vi "Save Waveform Results to CSV.vi"() -> ()   [LabVIEW 2010]
panel:
  out "error out":errorcluster
  in  "error in":errorcluster
  in  "results file":path=path "C:/Documents and Settings/user/Desktop/Claytons Archive/results.csv"
  in  "Data Files":path[](array[path])=[path "C:/5-01-003 Active Electrode Min Max/Waveform 1 -5 mA", path "C:/5-01-003 Active Electrode Min Max/Waveform 2 -0.02 mA", path "C:/5-01-003 Active Electrode Min Max/Waveform 3 -10 mA", path "C:/5-01-003 Active Electrode Min Max/Waveform 4 3 mA", path "C:/5-01-003 Active Electrode Min Max/Waveform 5 0.02 mA", path "C:/5-01-003 Active Electrode Min Max/Waveform 6 10 mA"]
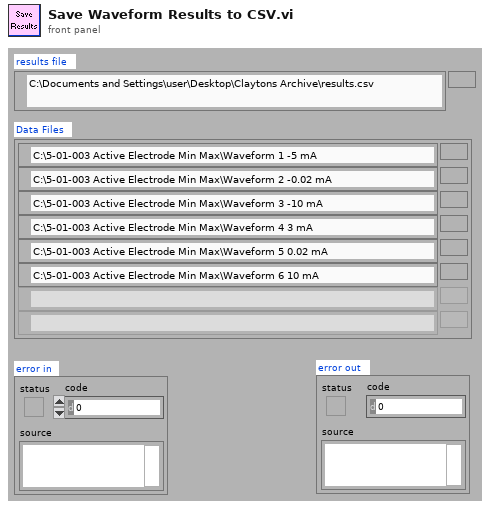
[diagram p1: front panel]
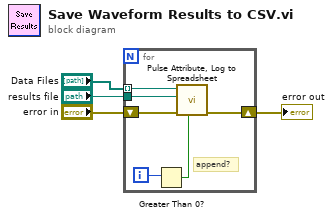
[diagram p0: block diagram]
diagram:
  n1 = for {
    shift-right: [w9] -> w2
    shift-left: "error in" -> [w10]
    tunnel: "Data Files" -> [w8] mode=indexing
    tunnel: "results file" -> [w7]
    i -> [w6]
    # "append?"
    n2 = Greater Than 0?(x=w6) -> (x > 0?=w5:bool)
    n3 = call "Pulse Attribute, Log to Spreadsheet.vi"("append to file (T)"=w5, "error in"=w10, "results file"=w7, "waveform file"=w8) -> ("error out"=w9:errorcluster)  [unwired: 5 in]
  }
  "error out" <- w2
